vi "Bit generator.vi"(0 "Bit":bool) -> ()   [LabVIEW 2017]
uses:
  <vilib>/eio/EIONode/EIONode.xnode
  <vilib>/rvi/eio/common/nirviEmuTemplateMethod_errors.vi
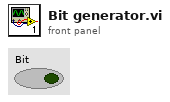
[diagram p1: front panel]
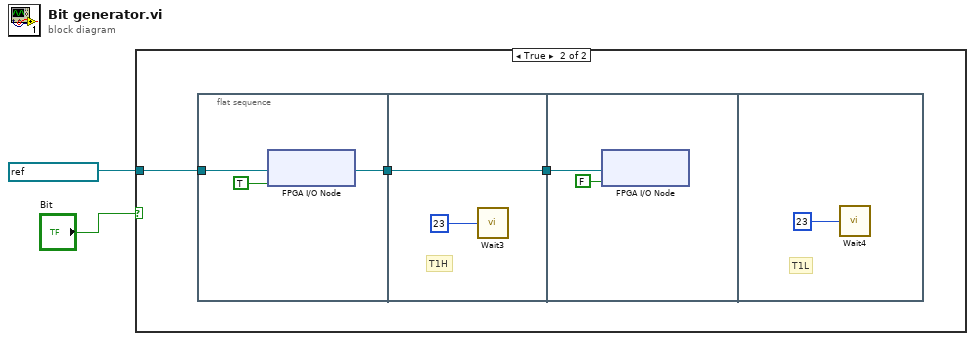
[diagram p0: block diagram]
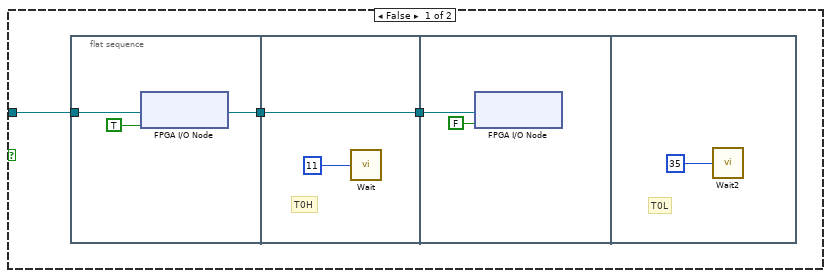
[diagram p2: hidden frame]
diagram:
  n1 = case shown="True" "Bit" {
    tunnel: refnum<k21> "Mod5/DIO1" ("FPGA I/O In") -> [w5 w16]
    frame False {
      n2 = flat-sequence {
        tunnel: w5 -> [w8]
        tunnel: [w6] -> w3
        tunnel: [w9] -> w4
        tunnel: w3 -> [w9]
        tunnel: w4 -> [w12]
        frame #0 {
          n3 = xnode "FPGA I/O Node"("I/O Item"=TRUE, "FPGA I/O In"=w8) -> ("FPGA I/O Out"=w6:refnum<k21>)
        }
        frame #1 {
          # "T0H"
          n4 = call "Wait"("Count(Ticks)"=u8 11) -> ()  [unwired: 1 out]
        }
        frame #2 {
          n5 = xnode "FPGA I/O Node"("I/O Item"=FALSE, "FPGA I/O In"=w12) -> ()  [unwired: 1 out]
        }
        frame #3 {
          # "T0L"
          n6 = call "Wait2"("Count(Ticks)"=u8 35) -> ()  [unwired: 1 out]
        }
      }
    }
    frame True {
      n7 = flat-sequence {
        tunnel: w16 -> [w19]
        tunnel: [w17] -> w14
        tunnel: [w20] -> w15
        tunnel: w14 -> [w20]
        tunnel: w15 -> [w23]
        frame #0 {
          n8 = xnode "FPGA I/O Node"("I/O Item"=TRUE, "FPGA I/O In"=w19) -> ("FPGA I/O Out"=w17:refnum<k21>)
        }
        frame #1 {
          # "T1H"
          n9 = call "Wait3"("Count(Ticks)"=u8 23) -> ()  [unwired: 1 out]
        }
        frame #2 {
          n10 = xnode "FPGA I/O Node"("I/O Item"=FALSE, "FPGA I/O In"=w23) -> ()  [unwired: 1 out]
        }
        frame #3 {
          # "T1L"
          n11 = call "Wait4"("Count(Ticks)"=u8 23) -> ()  [unwired: 1 out]
        }
      }
    }
  }
